vi "Get Marker Coordinates.vi"(8 "Coords 2":T1, 9 "Coords":T1, 10 "Type":T3, 11 "XYGraph in":refnum<vi>) -> (2 "Markers":T2, 3 "Cancelled":bool)   [LabVIEW 2020, in "Graph Extensions.lvlib"]
uses:
  Graph Extensions.lvlib
  controls/markerType.ctl
  controls/MarkerInfo.ctl
  <vilib>/Utility/miscctls.llb/LVPoint32TypeDef.ctl
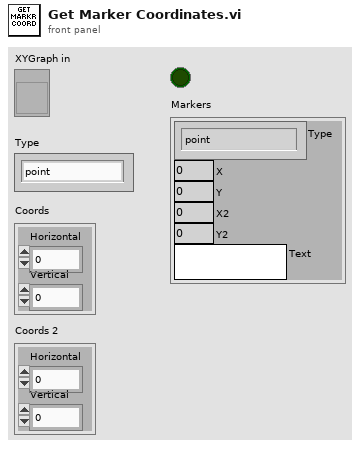
[diagram p1: front panel]
types:
  T1 = typedef "LVPoint32TypeDef.ctl" = cluster{"Horizontal":i32, "Vertical":i32}
  T2 = typedef "Graph Extensions.lvlib/MarkerInfo.ctl" = cluster{"Type":T3, "X":dbl, "Y":dbl, "X2":dbl, "Y2":dbl, "Text":string}
  T3 = typedef "Graph Extensions.lvlib/markerType.ctl" = enum16{"point", "arrow", "horiz", "vert", "vert range", "horiz range", "box"}
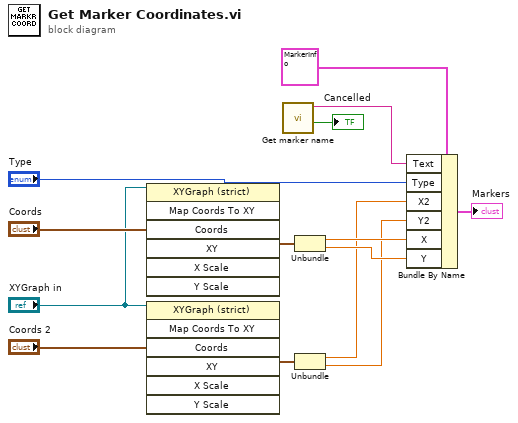
[diagram p0: block diagram]
diagram:
  n1 = invoke class="XYGraph (strict)" method="Map Coords To XY"(reference="XYGraph in", "Coords"="Coords") -> ("XY"=w11:cluster{"X":dbl, "Y":dbl})  [unwired: 5 in, 6 out]
  n2 = invoke class="XYGraph (strict)" method="Map Coords To XY"(reference="XYGraph in", "Coords"="Coords 2") -> ("XY"=w7:cluster{"X":dbl, "Y":dbl})  [unwired: 5 in, 6 out]
  n3 = call "Get marker name.vi"() -> ("cancelled"=→"Cancelled":bool, "text"=w2:string)  [unwired: 10 in]
  n4 = Unbundle(w11) -> ("X"=w6:dbl, "Y"=w5:dbl)
  n5 = Unbundle(w7) -> ("X"=w4:dbl, "Y"=w3:dbl)
  n6 = Bundle By Name(cluster=T2 {"Type"=enum."vert", "X"=2.0, "Y"=2.0, "X2"=2.0, "Y2"=2.0, "Text"="Drag and click to\nposition a marker"} ("Markers"), "Text"=w2, "Type"="Type", "X2"=w4, "Y2"=w3, "X"=w6, "Y"=w5) -> (→"Markers":T2)
